vi "parse_previous_series.vi"(8 "error in (no error)":errorcluster, 11 "MyComics.org_class in":refnum<class "MyComics.org_class.lvclass">) -> (0 "error out":errorcluster, 2 "prev seriesID":i32, 3 "MyComics.org_class out":refnum<class "MyComics.org_class.lvclass">)   [LabVIEW 2024, in "MyComics.org_class.lvclass"]
uses:
  MyComics.org_class.lvclass
  MyComics.org_class.lvclass/MyComics.org_class.ctl
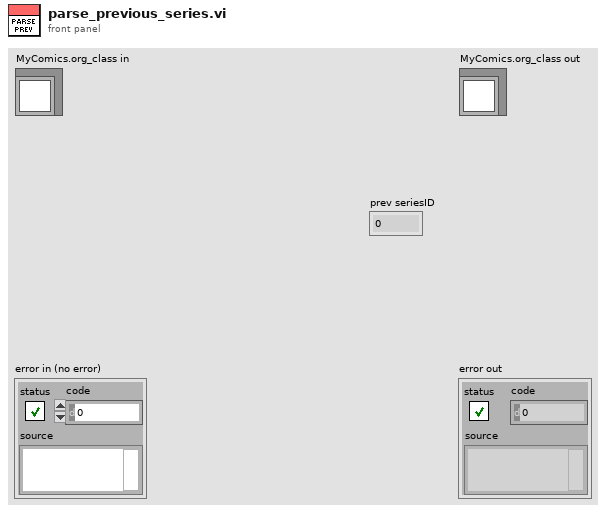
[diagram p1: front panel]
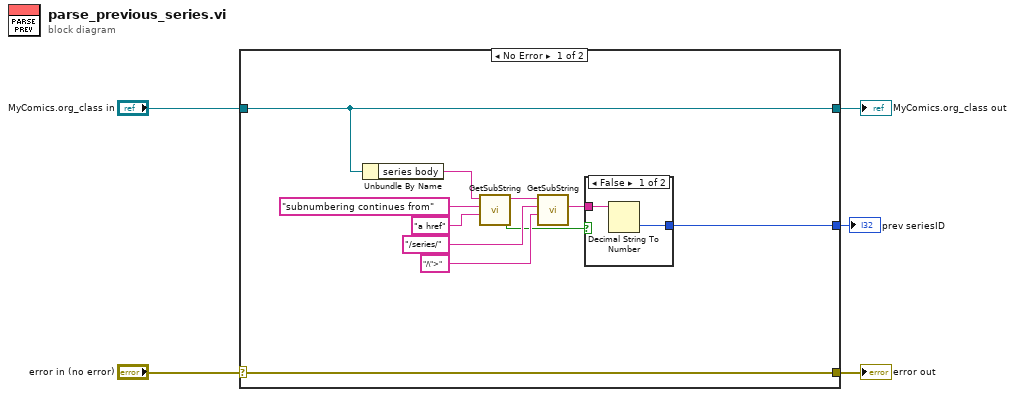
[diagram p0: block diagram]
diagram:
  n1 = case shown="No Error" "error in (no error)" {
    selector: "error in (no error)" -> [w16 w20]
    tunnel: [w16 w20] -> w4
    tunnel: [w15 w19] -> w2
    tunnel: "MyComics.org_class in" -> [w15 w19]
    tunnel: [w6 _] -> w1
    frame No Error {
      n2 = Unbundle By Name(w15) -> ("series body"=w7:string)
      n3 = call "GetSubString.vi"("End Search"="a href", "Start Search"="subnumbering continues from", "String In"=w7) -> ("Not Found?"=w8:bool, "Following String Out"=w12:string)  [unwired: 6 in, 1 out]
      n4 = call "GetSubString.vi"("End Search"="/\">" ("Start Search"), "Start Search"="/series/", "String In"=w12) -> ("Match"=w9:string)  [unwired: 6 in, 2 out]
      n5 = case shown="False" w8 {
        tunnel: w9 -> [w18 _]
        tunnel: [w17 _] -> w6
        frame False {
          n6 = Decimal String To Number(string=w18) -> (number=w17:i32)  [unwired: 2 in, 1 out]
        }
        frame True {
        }
      }
    }
    frame Error {
    }
  }
  "error out" <- w4
  "MyComics.org_class out" <- w2
  "prev seriesID" <- w1
